vi "Do Operation.vi"(10 "old":T1, 11 "Operation":T2) -> (2 "new":T1)   [LabVIEW 2022 SP3, in "AoC22.lvlib" / "Monkey.lvclass"]
uses:
  Monkey.lvclass
  Operation.ctl
  Op.ctl
  Worry Level.ctl
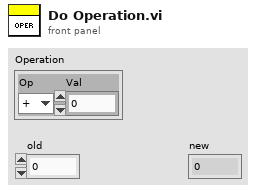
[diagram p1: front panel]
types:
  T1 = typedef "AoC22.lvlib/Monkey.lvclass/Worry Level.ctl" = u64
  T2 = typedef "AoC22.lvlib/Monkey.lvclass/Operation.ctl" = cluster{"Op":T3, "Val":T1}
  T3 = typedef "AoC22.lvlib/Monkey.lvclass/Op.ctl" = enum16{"+", "*"}
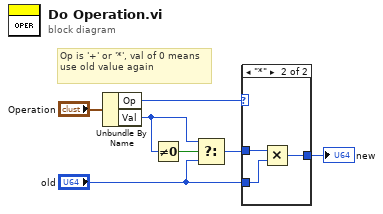
[diagram p0: block diagram]
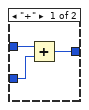
[diagram p2: hidden frame]
diagram:
  # "Op is '+' or '*', val of 0 means use old value again"
  n1 = Unbundle By Name("Operation") -> ("Op"=w2:T3, "Val"=w5:T1)
  n2 = Not Equal To 0?(x=w5) -> (x != 0?=w6:bool)
  n3 = Select(t=w5, s=w6, f="old") -> (s? t:f=w3:T1)
  n4 = case shown="\"*\"" w2 {
    tunnel: "old" -> [w9 w12]
    tunnel: w3 -> [w10 w13]
    tunnel: [w8 w11] -> w1
    frame "+" {
      n5 = Add(x=w10, y=w9) -> (x+y=w8:T1)
    }
    frame "*" {
      n6 = Multiply(x=w13, y=w12) -> (x*y=w11:T1)
    }
  }
  "new" <- w1
